vi "isSet.vi"(9 "Error":dbl, 10 "Current Value":dbl, 11 "Setpoint":dbl) -> (3 "Finished":bool)   [LabVIEW 2015]
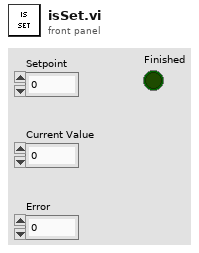
[diagram p1: front panel]
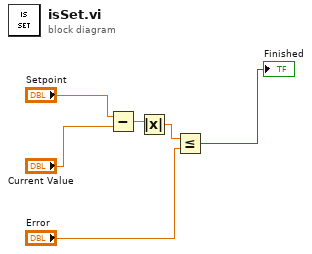
[diagram p0: block diagram]
diagram:
  n1 = Subtract(x="Setpoint", y="Current Value") -> (x-y=w4:dbl)
  n2 = Absolute Value(x=w4) -> (abs(x)=w3:dbl)
  n3 = Less Or Equal?(x=w3, y="Error") -> (x <= y?=→"Finished":bool)
